vi "Generic I2C RX Config.vi"(8 "error in (no error)":errorcluster, 11 "Generic I2C.lvclass In":refnum<class "Generic I2C.lvclass">) -> (0 "error out":errorcluster, 3 "Generic I2C.lvclass Out":refnum<class "Generic I2C.lvclass">)   [LabVIEW 2020, in "Generic I2C.lvlib" / "Simulation.lvclass"]
uses:
  Simulation.lvclass
  Parent/Generic I2C.lvclass
  C:/Users/kaiser.asan/OneDrive - SolitonTechnologies/LabVIEW/29.SDLC - I2C Driver/I2C Module/I2C Controller Module/Class/Devices/Parent/Devices.lvclass
panel:
  in  "Save?":bool caption="Save Button"
  in  "RX.Data":u8[](array[numeric]) caption="Read Bytes" format="%.0x"
  # "Target Configuration"
  # "Enter the data to be sent back by the Target"
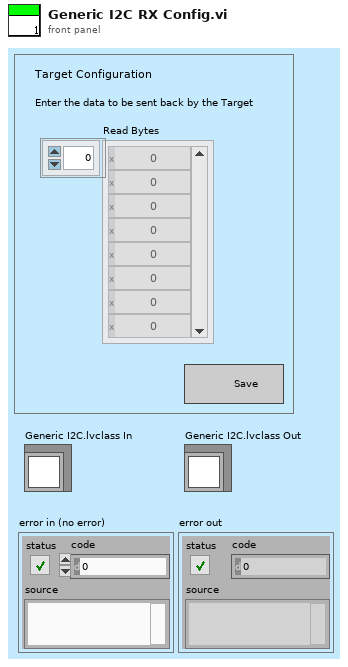
[diagram p1: front panel]
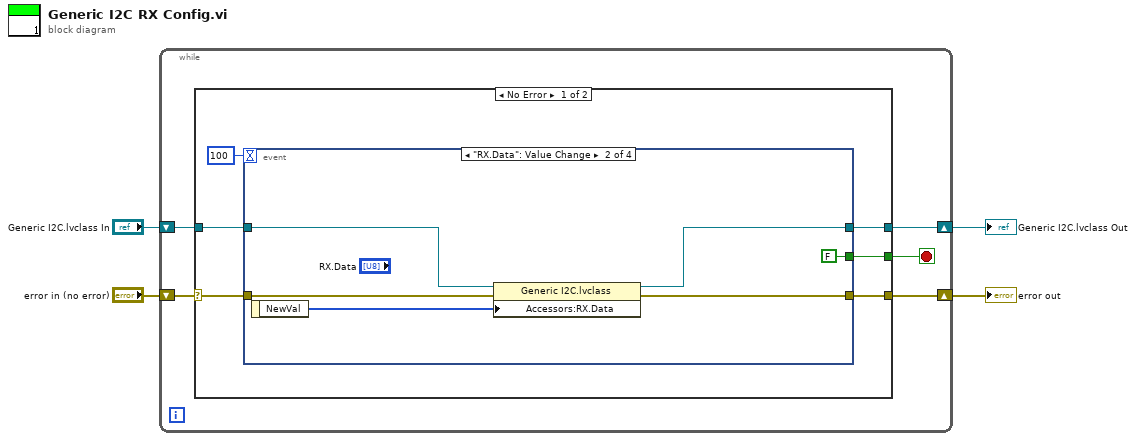
[diagram p0: block diagram]
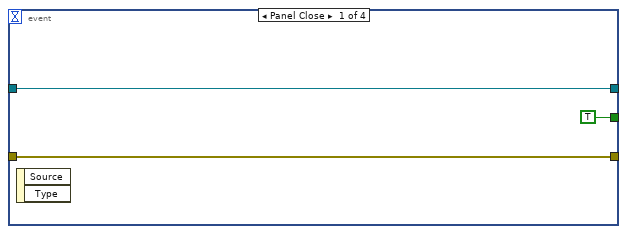
[diagram p2: hidden frame]
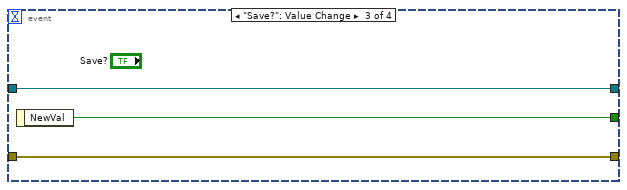
[diagram p3: hidden frame]
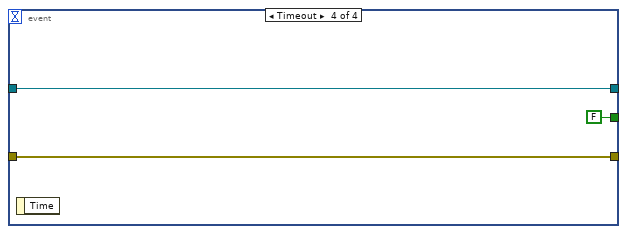
[diagram p4: hidden frame]
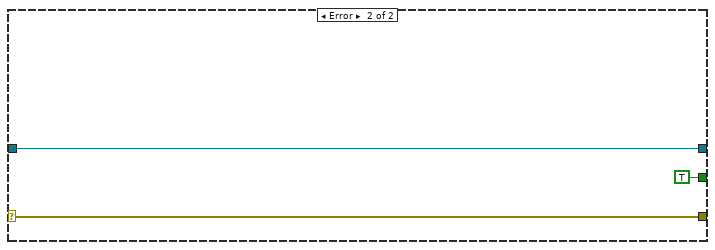
[diagram p5: hidden frame]
diagram:
  n1 = while {
    shift-right: [w9] -> w3
    shift-left: "error in (no error)" -> [w8]
    shift-right: [w6] -> w2
    shift-left: "Generic I2C.lvclass In" -> [w7]
    stop <- w5 stop-if-true
    n2 = case shown="No Error" w8 {
      selector: w8 -> [w14 w31]
      tunnel: [w15 w31] -> w9
      tunnel: w7 -> [w13 w32]
      tunnel: [w12 w32] -> w6
      tunnel: [w11 TRUE ("NewVal")] -> w5
      frame No Error {
        n3 = event shown="[1] \"RX.Data\": Value Change" {
          selector: _ -> [_ _ _ _]
          dyn-events: _ -> [_ _ _ _]
          timeout: 100 -> [_ _ _ _]
          tunnel: [w18 w23 w27 w30] -> w15
          tunnel: w14 -> [w18 w24 w27 w30]
          tunnel: w13 -> [w16 w21 w25 w29]
          tunnel: [w16 w20 w25 w29] -> w12
          tunnel: [TRUE FALSE ("NewVal") w26 FALSE ("NewVal")] -> w11
          event Panel Close {
            n4 = event-data() -> ()  [unwired: 1 in, 2 out]
          }
          event "RX.Data": Value Change {
            n5 = event-data() -> ("NewVal"=w22:u8[])  [unwired: 1 in]
            n6 = property class="Generic I2C.lvclass"(reference=w21, error in=w24, "Accessors:RX.Data"=w22) -> (reference out=w20:refnum<class "Generic I2C.lvclass">, error out=w23:errorcluster)
          }
          event "Save?": Value Change {
            n7 = event-data() -> ("NewVal"=w26:bool)  [unwired: 1 in]
          }
          event Timeout {
            n8 = event-data() -> ()  [unwired: 1 in, 1 out]
          }
        }
      }
      frame Error {
      }
    }
  }
  "error out" <- w3
  "Generic I2C.lvclass Out" <- w2
